vi "From String Array.vi"(8 "error in (no error)":errorcluster, 9 "String Array":string[](array[string]), 11 "Wait Step Config in":refnum<class "Wait Step Config.lvclass">) -> (0 "error out":errorcluster, 3 "Wait Step Config out":refnum<class "Wait Step Config.lvclass">)   [LabVIEW 2015, in "Wait Step Config.lvclass"]
uses:
  Wait Step Config.lvclass
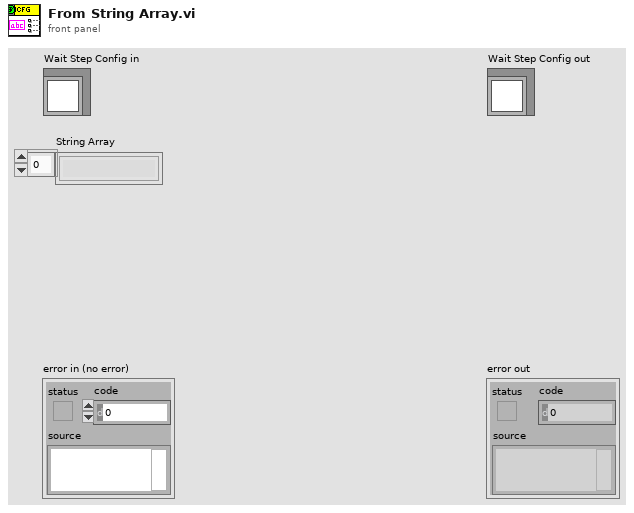
[diagram p1: front panel]
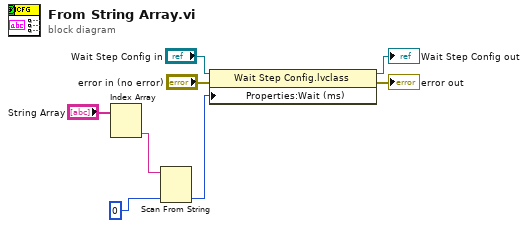
[diagram p0: block diagram]
diagram:
  n1 = Index Array(array="String Array") -> (element #2=w1:string)  [unwired: 2 in, 1 out]
  n2 = Scan From String(input string=w1, default 1=u32 0 ("Wait (ms)")) -> (output 1=w2:u32)  [unwired: 3 in, 3 out]
  n3 = property class="Wait Step Config.lvclass"(reference="Wait Step Config in", error in="error in (no error)", "Properties:Wait (ms)"=w2) -> (reference out=→"Wait Step Config out":refnum<class "Wait Step Config.lvclass">, error out=→"error out":errorcluster)
